vi "Connect.vi"(8 "error in (no error)":errorcluster, 11 "PLCHandler in":refnum<class "PLCHandler.lvclass">) -> (0 "error out":errorcluster, 3 "PLCHandler out":refnum<class "PLCHandler.lvclass">)   [LabVIEW 2022 SP3, in "PLCHandler.lvlib" / "PLCHandler.lvclass"]
uses:
  PLCHandler.lvclass
  PLCHandler.lvclass/PLCHandler.ctl
  <vilib>/NI/Modbus Library/API/Wrapper/Create Serial Master.vi
  <vilib>/NI/Modbus Library/API/Wrapper/API Main.lvlib
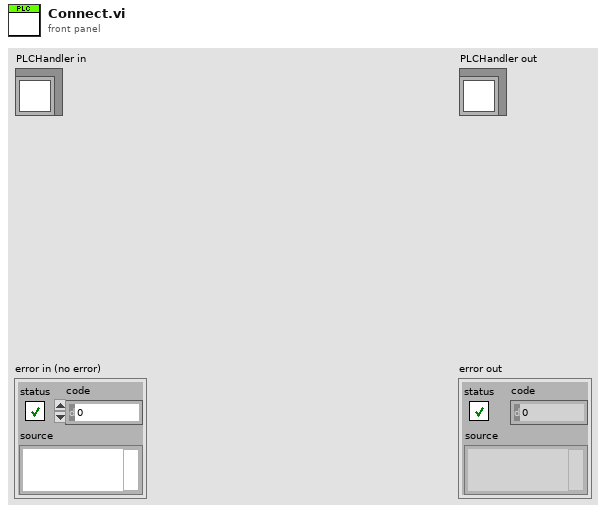
[diagram p1: front panel]
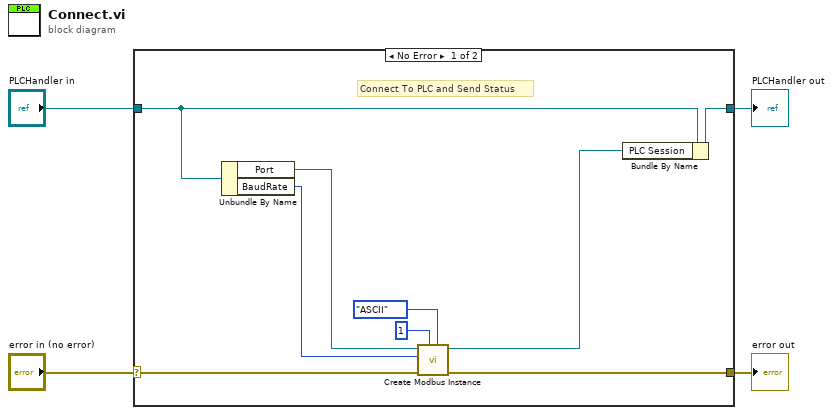
[diagram p0: block diagram]
diagram:
  n1 = case shown="No Error" "error in (no error)" {
    selector: "error in (no error)" -> [w13 w15]
    tunnel: [w11 w15] -> w3
    tunnel: [w6 w14] -> w1
    tunnel: "PLCHandler in" -> [w12 w14]
    frame No Error {
      # "Connect To PLC and Send Status"
      n2 = Unbundle By Name(w12) -> ("Port"=w10:refnum<visa-resource-name>, "BaudRate"=w9:u32)
      n3 = call-poly <vilib>:"Create Modbus Instance.vi"("serial type"=enum16{"RTU", "ASCII"}."ASCII", "unit ID"=u8 1, "error in"=w13, "baud rate"=w9, "VISA resource name"=w10) -> ("error out"=w11:errorcluster, "serial master instance"=w5:refnum<class "Modbus Master.lvclass">)  [unwired: 5 in]
      n4 = Bundle By Name(cluster=w12, "PLC Session"=w5) -> (w6:refnum<class "PLCHandler.lvclass">)
    }
    frame Error {
    }
  }
  "error out" <- w3
  "PLCHandler out" <- w1
